vi "ControlShooter.vi"(1 "State":T2) -> (0 "To Shooter\nSolenoid Loop":T1=enum."Forward")   [LabVIEW 2013]
uses:
  typedefs/subStates.ctl
  <vilib>/Rock Robotics/WPI/Solenoid/WPI_SolenoidValue.ctl
  typedefs/fg_typedef.ctl
  <vilib>/Rock Robotics/WPI/Solenoid/WPI_SolenoidGetEnum.vi
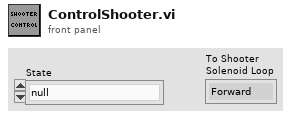
[diagram p1: front panel]
types:
  T1 = typedef "WPI_SolenoidValue.ctl" = enum16{"Off", "On", "Forward", "Reverse"}
  T2 = typedef "subStates.ctl" = enum16{"null", "wait", "driver control", "auto", "manual override", "hold position", "rotate", "pickup", "pass", "load", "goto shoot", "shoot", "cancel", "end"}
  T3 = typedef "fg_typedef.ctl" = enum16{"Get", "Set"}
  T4 = typedef "WPI_DigitalInputDevRef.ctl" = cluster{"DevStatus":errorcluster, "DIO Channel":T5, "Digital Module":T6}
  T5 = typedef "FPGA_DIOChannel.ctl" = enum8{"DIO 1", "DIO 2", "DIO 3", "DIO 4", "DIO 5", "DIO 6", "DIO 7", "DIO 8", "DIO 9", "DIO 10", "DIO 11", "DIO 12", "DIO 13", "DIO 14", "Invalid"}
  T6 = typedef "FPGA_TypedefDigitalModule.ctl" = enum16{"Digital Module 1", "Digital Module 2"}
  T7 = typedef "WPI_SolenoidDevRef.ctl" = cluster{"DevStatus":errorcluster, "Solenoid Module":T8, "Forward Solenoid Channel":T9, "Reverse Solenoid Channel":T9}
  T8 = typedef "FPGA_TypedefSolenoidModule.ctl" = enum16{"Solenoid Module 1", "Solenoid Module 2"}
  T9 = typedef "WPI_SolenoidChannel.ctl" = enum8{"Solenoid 1", "Solenoid 2", "Solenoid 3", "Solenoid 4", "Solenoid 5", "Solenoid 6", "Solenoid 7", "Solenoid 8", "Invalid"}
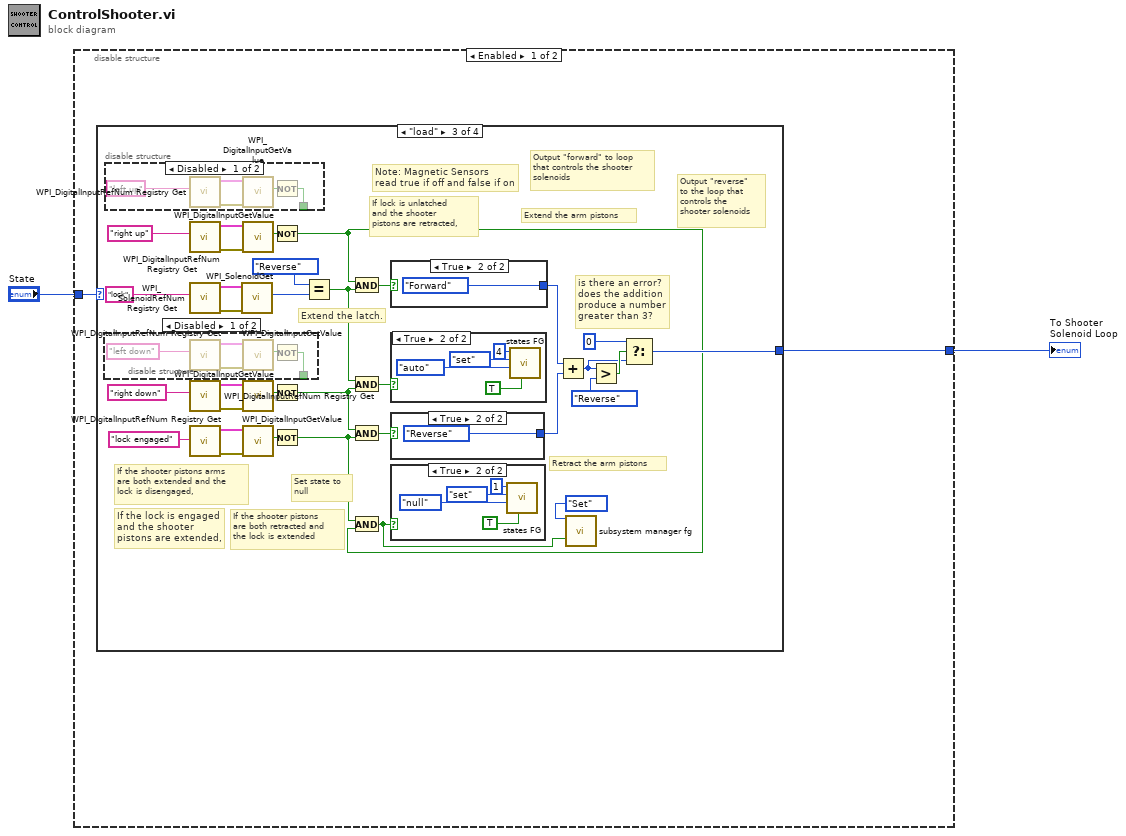
[diagram p0: block diagram]
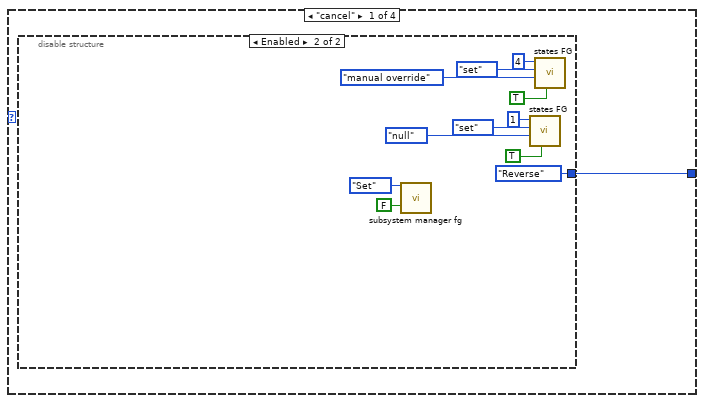
[diagram p2: hidden frame]
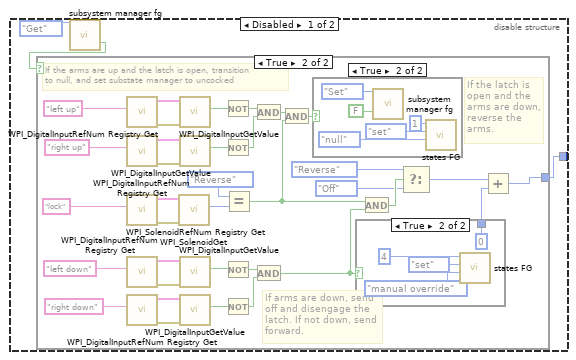
[diagram p3: hidden frame]
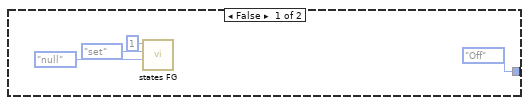
[diagram p4: hidden frame]
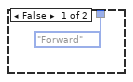
[diagram p6: hidden frame]
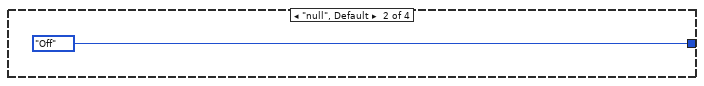
[diagram p7: hidden frame]
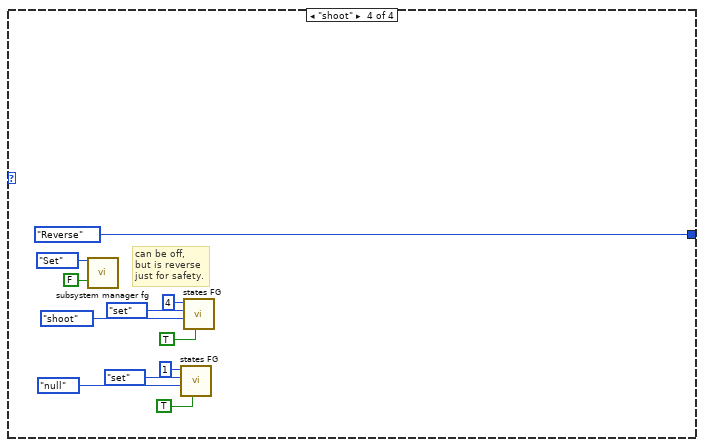
[diagram p14: hidden frame]
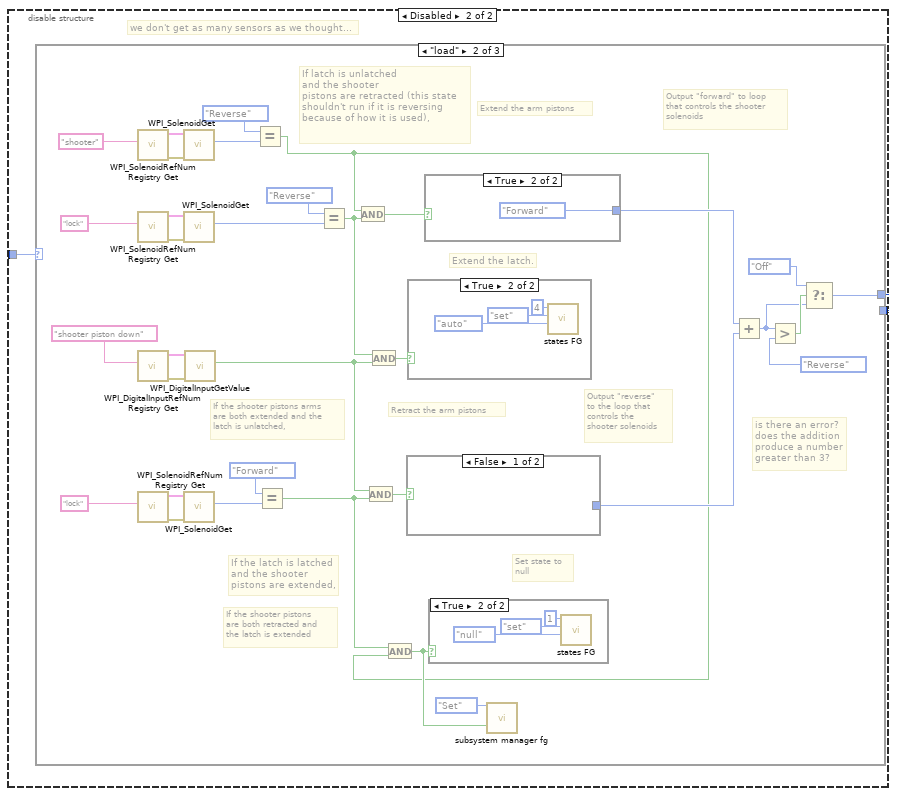
[diagram p15: hidden frame]
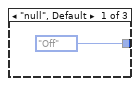
[diagram p16: hidden frame]
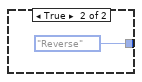
[diagram p18: hidden frame]
diagram:
  n1 = disable-structure shown="Enabled" {
    disable-tunnel: "State" -> [w4 w135]
    disable-tunnel: [w3 w134] -> w1
    frame Enabled {
      n2 = case shown="\"load\"" w4 {
        tunnel: [w5 WPI_SolenoidValue."Off" ("To Shooter\nSolenoid Loop") w82 WPI_SolenoidValue."Reverse" ("To Shooter\nSolenoid Loop")] -> w3
        frame "cancel" {
          n3 = disable-structure shown="Enabled" {
            disable-tunnel: [w6 WPI_SolenoidValue."Reverse" ("To Shooter\nSolenoid Loop")] -> w5
            frame Disabled {
              n4 = call "subsystem manager fg.vi"("Menu"=fg_typedef."Get") -> ("Shooter Cocked"=w7:bool)  [unwired: 14 in, 4 out]
              n5 = case shown="True" w7 {
                tunnel: [WPI_SolenoidValue."Off" ("To Shooter\nSolenoid Loop") w16] -> w6
                frame False {
                  n6 = call "states FG.vi"("subState in"=subStates."null", "menu (get)"=enum16{"set", "get"}."set", "Loop ID"=1) -> ()  [unwired: 5 in, 4 out]
                }
                frame True {
                  # "If the arms are up and the latch is open, transition\nto null, and set substate manager to uncocked"
                  # "If the latch is\nopen and the\narms are down,\nreverse the\narms."
                  # "If arms are down, send\noff and disengage the\nlatch. If not down, send\nforward."
                  n7 = call <vilib>:"WPI_DigitalInputRefNum Registry Get.vi"("refnum name"="left up") -> ("error out"=w34:errorcluster, "DigitalInputDevRef"=w33:T4)  [unwired: 9 in]
                  n8 = call <vilib>:"WPI_DigitalInputRefNum Registry Get.vi"("refnum name"="right up") -> ("error out"=w31:errorcluster, "DigitalInputDevRef"=w30:T4)  [unwired: 9 in]
                  n9 = call <vilib>:"WPI_SolenoidRefNum Registry Get.vi"("refnum name"="lock") -> ("error out"=w27:errorcluster, "SolenoidDevRef"=w28:T7)  [unwired: 9 in]
                  n10 = call <vilib>:"WPI_DigitalInputRefNum Registry Get.vi"("refnum name"="left down") -> ("error out"=w37:errorcluster, "DigitalInputDevRef"=w36:T4)  [unwired: 9 in]
                  n11 = call <vilib>:"WPI_DigitalInputRefNum Registry Get.vi"("refnum name"="right down") -> ("error out"=w40:errorcluster, "DigitalInputDevRef"=w39:T4)  [unwired: 9 in]
                  n12 = call-poly <vilib>:"WPI_SolenoidGet.vi"("error in (no error)"=w27, "SolenoidDevRef"=w28) -> ("Value"=w46:T1)  [unwired: 7 in, 2 out]
                  n13 = call <vilib>:"WPI_DigitalInputGetValue.vi"("error in (no error)"=w34, "DigitalInputDevRef"=w33) -> ("Value"=w45:bool)  [unwired: 7 in, 2 out]
                  n14 = call <vilib>:"WPI_DigitalInputGetValue.vi"("error in (no error)"=w31, "DigitalInputDevRef"=w30) -> ("Value"=w44:bool)  [unwired: 7 in, 2 out]
                  n15 = call <vilib>:"WPI_DigitalInputGetValue.vi"("error in (no error)"=w37, "DigitalInputDevRef"=w36) -> ("Value"=w43:bool)  [unwired: 7 in, 2 out]
                  n16 = call <vilib>:"WPI_DigitalInputGetValue.vi"("error in (no error)"=w40, "DigitalInputDevRef"=w39) -> ("Value"=w42:bool)  [unwired: 7 in, 2 out]
                  n17 = Not(x=w45) -> (.not. x?=w25:bool)
                  n18 = Not(x=w44) -> (.not. x?=w26:bool)
                  n19 = Not(x=w43) -> (.not. x?=w23:bool)
                  n20 = Not(x=w42) -> (.not. x?=w24:bool)
                  n21 = Equal?(x=WPI_SolenoidValue."Reverse", y=w46) -> (x = y?=w14:bool)
                  n22 = And(x=w25, y=w26) -> (x .and. y?=w15:bool)
                  n23 = And(x=w23, y=w24) -> (x .and. y?=w22:bool)
                  n24 = And(x=w15, y=w14) -> (x .and. y?=w13:bool)
                  n25 = case shown="True" w13 {
                    frame False {
                    }
                    frame True {
                      n26 = call "subsystem manager fg.vi"("Menu"=fg_typedef."Set", "Shooter Cocked"=FALSE) -> ()  [unwired: 13 in, 5 out]
                      n27 = call "states FG.vi"("subState in"=subStates."null", "menu (get)"=enum16{"set", "get"}."set", "Loop ID"=1) -> ()  [unwired: 5 in, 4 out]
                    }
                  }
                  n28 = case shown="True" w22 {
                    tunnel: [WPI_SolenoidValue."Forward" ("To Shooter\nSolenoid Loop") 0] -> w21
                    frame False {
                    }
                    frame True {
                      n29 = call "states FG.vi"("subState in"=subStates."manual override", "menu (get)"=enum16{"set", "get"}."set", "Loop ID"=4) -> ()  [unwired: 5 in, 4 out]
                    }
                  }
                  n30 = And(x=w14, y=w22) -> (x .and. y?=w20:bool)
                  n31 = Select(t=WPI_SolenoidValue."Reverse" ("To Shooter\nSolenoid Loop"), s=w20, f=WPI_SolenoidValue."Off") -> (s? t:f=w18:T1)
                  n32 = Add(x=w18, y=w21) -> (x+y=w16:i32)
                }
              }
            }
            frame Enabled {
              n33 = call "subsystem manager fg.vi"("Menu"=fg_typedef."Set", "Shooter Cocked"=FALSE) -> ()  [unwired: 13 in, 5 out]
              n34 = call "states FG.vi"("exit in"=TRUE, "subState in"=subStates."null", "menu (get)"=enum16{"set", "get"}."set", "Loop ID"=1) -> ()  [unwired: 4 in, 4 out]
              n35 = call "states FG.vi"("exit in"=TRUE, "subState in"=subStates."manual override", "menu (get)"=enum16{"set", "get"}."set", "Loop ID"=4) -> ()  [unwired: 4 in, 4 out]
            }
          }
        }
        frame "null", Default {
        }
        frame "load" {
          # "Note: Magnetic Sensors\nread true if off and false if on"
          # "is there an error?\ndoes the addition\nproduce a number \ngreater than 3?"
          # "Output \"reverse\"\nto the loop that\ncontrols the\nshooter solenoids"
          # "Output \"forward\" to loop\nthat controls the shooter\nsolenoids"
          # "Set state to\nnull"
          # "If the shooter pistons\nare both retracted and\nthe lock is extended"
          # "If the lock is engaged\nand the shooter\npistons are extended,"
          # "Retract the arm pistons"
          # "If lock is unlatched\nand the shooter\npistons are retracted,"
          # "Extend the latch."
          # "If the shooter pistons arms\nare both extended and the\nlock is disengaged,"
          # "Extend the arm pistons"
          n36 = disable-structure shown="Disabled" {
            disable-tunnel: [w103 _] -> _
            frame Disabled {
              n37 = call <vilib>:"WPI_DigitalInputRefNum Registry Get.vi"("refnum name"="left down") -> ("error out"=w106:errorcluster, "DigitalInputDevRef"=w107:T4)  [unwired: 9 in]
              n38 = call <vilib>:"WPI_DigitalInputGetValue.vi"("error in (no error)"=w106, "DigitalInputDevRef"=w107) -> ("Value"=w104:bool)  [unwired: 7 in, 2 out]
              n39 = Not(x=w104) -> (.not. x?=w103:bool)
            }
            frame Enabled {
            }
          }
          n40 = disable-structure shown="Disabled" {
            disable-tunnel: [w108 _] -> _
            frame Disabled {
              n41 = call <vilib>:"WPI_DigitalInputRefNum Registry Get.vi"("refnum name"="left up") -> ("error out"=w111:errorcluster, "DigitalInputDevRef"=w112:T4)  [unwired: 9 in]
              n42 = call <vilib>:"WPI_DigitalInputGetValue.vi"("error in (no error)"=w111, "DigitalInputDevRef"=w112) -> ("Value"=w109:bool)  [unwired: 7 in, 2 out]
              n43 = Not(x=w109) -> (.not. x?=w108:bool)
            }
            frame Enabled {
            }
          }
          n44 = call <vilib>:"WPI_DigitalInputRefNum Registry Get.vi"("refnum name"="right up") -> ("error out"=w96:errorcluster, "DigitalInputDevRef"=w97:T4)  [unwired: 9 in]
          n45 = call <vilib>:"WPI_SolenoidRefNum Registry Get.vi"("refnum name"="lock") -> ("error out"=w102:errorcluster, "SolenoidDevRef"=w101:T7)  [unwired: 9 in]
          n46 = call <vilib>:"WPI_DigitalInputRefNum Registry Get.vi"("refnum name"="right down") -> ("error out"=w91:errorcluster, "DigitalInputDevRef"=w92:T4)  [unwired: 9 in]
          n47 = call <vilib>:"WPI_DigitalInputRefNum Registry Get.vi"("refnum name"="lock engaged") -> ("error out"=w76:errorcluster, "DigitalInputDevRef"=w77:T4)  [unwired: 9 in]
          n48 = call-poly <vilib>:"WPI_SolenoidGet.vi"("error in (no error)"=w102, "SolenoidDevRef"=w101) -> ("Value"=w99:T1)  [unwired: 7 in, 2 out]
          n49 = call <vilib>:"WPI_DigitalInputGetValue.vi"("error in (no error)"=w96, "DigitalInputDevRef"=w97) -> ("Value"=w72:bool)  [unwired: 7 in, 2 out]
          n50 = call <vilib>:"WPI_DigitalInputGetValue.vi"("error in (no error)"=w91, "DigitalInputDevRef"=w92) -> ("Value"=w73:bool)  [unwired: 7 in, 2 out]
          n51 = call <vilib>:"WPI_DigitalInputGetValue.vi"("error in (no error)"=w76, "DigitalInputDevRef"=w77) -> ("Value"=w75:bool)  [unwired: 7 in, 2 out]
          n52 = Not(x=w72) -> (.not. x?=w71:bool)
          n53 = Not(x=w73) -> (.not. x?=w70:bool)
          n54 = Not(x=w75) -> (.not. x?=w74:bool)
          n55 = Equal?(x=WPI_SolenoidValue."Reverse", y=w99) -> (x = y?=w88:bool)
          n56 = And(x=w71, y=w88) -> (x .and. y?=w94:bool)
          n57 = And(x=w88, y=w70) -> (x .and. y?=w93:bool)
          n58 = And(x=w70, y=w74) -> (x .and. y?=w89:bool)
          n59 = And(x=w74, y=w71) -> (x .and. y?=w79:bool)
          n60 = case shown="True" w94 {
            tunnel: [_ WPI_SolenoidValue."Forward" ("Value")] -> w87
            frame False {
            }
            frame True {
            }
          }
          n61 = case shown="True" w93 {
            frame False {
            }
            frame True {
              n62 = call "states FG.vi"("exit in"=TRUE, "subState in"=subStates."auto", "menu (get)"=enum16{"set", "get"}."set", "Loop ID"=4) -> ()  [unwired: 4 in, 4 out]
            }
          }
          n63 = case shown="True" w89 {
            tunnel: [_ WPI_SolenoidValue."Reverse" ("Value")] -> w81
            frame False {
            }
            frame True {
            }
          }
          n64 = case shown="True" w79 {
            frame False {
            }
            frame True {
              n65 = call "states FG.vi"("exit in"=TRUE, "subState in"=subStates."null", "menu (get)"=enum16{"set", "get"}."set", "Loop ID"=1) -> ()  [unwired: 4 in, 4 out]
            }
          }
          n66 = Add(x=w87, y=w81) -> (x+y=w84:u16)
          n67 = call "subsystem manager fg.vi"("Menu"=fg_typedef."Set", "Shooter Cocked"=w79) -> ()  [unwired: 13 in, 5 out]
          n68 = Greater?(x=w84, y=WPI_SolenoidValue."Reverse" ("Value")) -> (0:w85:bool)
          n69 = Select(t=0, s=w85, f=w84) -> (s? t:f=w82:i32)
        }
        frame "shoot" {
          # "can be off,\nbut is reverse\njust for safety."
          n70 = call "subsystem manager fg.vi"("Menu"=fg_typedef."Set", "Shooter Cocked"=FALSE) -> ()  [unwired: 13 in, 5 out]
          n71 = call "states FG.vi"("exit in"=TRUE, "subState in"=subStates."null", "menu (get)"=enum16{"set", "get"}."set", "Loop ID"=1) -> ()  [unwired: 4 in, 4 out]
          n72 = call "states FG.vi"("exit in"=TRUE, "subState in"=subStates."shoot", "menu (get)"=enum16{"set", "get"}."set", "Loop ID"=4) -> ()  [unwired: 4 in, 4 out]
        }
      }
    }
    frame Disabled {
      # "we don't get as many sensors as we thought..."
      n73 = case shown="\"load\"" w135 {
        tunnel: [WPI_SolenoidValue."Off" ("To Shooter\nSolenoid Loop") w148 WPI_SolenoidValue."Off" ("To Shooter\nSolenoid Loop")] -> w134
        frame "null", Default {
        }
        frame "load" {
          # "is there an error?\ndoes the addition\nproduce a number \ngreater than 3?"
          # "Output \"reverse\"\nto the loop that\ncontrols the\nshooter solenoids"
          # "Output \"forward\" to loop\nthat controls the shooter\nsolenoids"
          # "Set state to\nnull"
          # "If the shooter pistons\nare both retracted and\nthe latch is extended"
          # "If the latch is latched\nand the shooter\npistons are extended,"
          # "Retract the arm pistons"
          # "If latch is unlatched\nand the shooter\npistons are retracted (this state shouldn't run if it is reversing because of how it is used),"
          # "Extend the latch."
          # "If the shooter pistons arms\nare both extended and the\nlatch is unlatched,"
          # "Extend the arm pistons"
          n74 = call <vilib>:"WPI_SolenoidRefNum Registry Get.vi"("refnum name"="shooter") -> ("error out"=w140:errorcluster, "SolenoidDevRef"=w141:T7)  [unwired: 9 in]
          n75 = call <vilib>:"WPI_SolenoidRefNum Registry Get.vi"("refnum name"="lock") -> ("error out"=w170:errorcluster, "SolenoidDevRef"=w169:T7)  [unwired: 9 in]
          n76 = call <vilib>:"WPI_DigitalInputRefNum Registry Get.vi"("refnum name"="shooter piston down") -> ("error out"=w162:errorcluster, "DigitalInputDevRef"=w163:T4)  [unwired: 9 in]
          n77 = call <vilib>:"WPI_SolenoidRefNum Registry Get.vi"("refnum name"="lock") -> ("error out"=w160:errorcluster, "SolenoidDevRef"=w159:T7)  [unwired: 9 in]
          n78 = call-poly <vilib>:"WPI_SolenoidGet.vi"("error in (no error)"=w140, "SolenoidDevRef"=w141) -> ("Value"=w142:T1)  [unwired: 7 in, 2 out]
          n79 = call-poly <vilib>:"WPI_SolenoidGet.vi"("error in (no error)"=w170, "SolenoidDevRef"=w169) -> ("Value"=w167:T1)  [unwired: 7 in, 2 out]
          n80 = call-poly <vilib>:"WPI_SolenoidGet.vi"("error in (no error)"=w160, "SolenoidDevRef"=w159) -> ("Value"=w157:T1)  [unwired: 7 in, 2 out]
          n81 = call <vilib>:"WPI_DigitalInputGetValue.vi"("error in (no error)"=w162, "DigitalInputDevRef"=w163) -> ("Value"=w144:bool)  [unwired: 7 in, 2 out]
          n82 = Equal?(x=WPI_SolenoidValue."Reverse", y=w142) -> (x = y?=w138:bool)
          n83 = Equal?(x=WPI_SolenoidValue."Forward", y=w157) -> (x = y?=w153:bool)
          n84 = Equal?(x=WPI_SolenoidValue."Reverse", y=w167) -> (x = y?=w154:bool)
          n85 = And(x=w138, y=w154) -> (x .and. y?=w165:bool)
          n86 = And(x=w144, y=w153) -> (x .and. y?=w155:bool)
          n87 = And(x=w154, y=w144) -> (x .and. y?=w164:bool)
          n88 = And(x=w153, y=w138) -> (x .and. y?=w145:bool)
          n89 = case shown="False" w155 {
            tunnel: [_ WPI_SolenoidValue."Reverse" ("Value")] -> w147
            frame False {
            }
            frame True {
            }
          }
          n90 = case shown="True" w164 {
            frame False {
            }
            frame True {
              n91 = call "states FG.vi"("subState in"=subStates."auto", "menu (get)"=enum16{"set", "get"}."set", "Loop ID"=4) -> ()  [unwired: 5 in, 4 out]
            }
          }
          n92 = case shown="True" w165 {
            tunnel: [_ WPI_SolenoidValue."Forward" ("Value")] -> w152
            frame False {
            }
            frame True {
            }
          }
          n93 = case shown="True" w145 {
            frame False {
            }
            frame True {
              n94 = call "states FG.vi"("subState in"=subStates."null", "menu (get)"=enum16{"set", "get"}."set", "Loop ID"=1) -> ()  [unwired: 5 in, 4 out]
            }
          }
          n95 = call "subsystem manager fg.vi"("Menu"=fg_typedef."Set", "Shooter Cocked"=w145) -> ()  [unwired: 13 in, 5 out]
          n96 = Add(x=w152, y=w147) -> (x+y=w149:u16)
          n97 = Greater?(x=w149, y=WPI_SolenoidValue."Reverse" ("Value")) -> (0:w150:bool)
          n98 = Select(t=WPI_SolenoidValue."Off" ("Value"), s=w150, f=w149) -> (s? t:f=w148:u16)
        }
        frame "shoot" {
          n99 = call "states FG.vi"("subState in"=subStates."null", "menu (get)"=enum16{"set", "get"}."set", "Loop ID"=1) -> ()  [unwired: 5 in, 4 out]
          n100 = call "states FG.vi"("subState in"=subStates."shoot", "menu (get)"=enum16{"set", "get"}."set", "Loop ID"=4) -> ()  [unwired: 5 in, 4 out]
        }
      }
    }
  }
  "To Shooter\nSolenoid Loop" <- w1
